vi "Lookup (Wfm Data Ref).vi"(8 "error in (no error)":errorcluster, 10 "Wfm Data Ref":T1, 11 "Reference Dictionary in":refnum<class "Reference Dictionary.lvclass">) -> (0 "error out":errorcluster, 1 "Index":i32, 2 "Found":bool, 3 "Reference Dictionary out":refnum<class "Reference Dictionary.lvclass">)   [LabVIEW 2015, in "Reference Dictionary.lvclass"]
uses:
  Reference Dictionary.lvclass
  <vilib>/NI Veristand/Custom Device API/Waveform Data Reference.ctl
  Reference Dictionary.lvclass/Reference Dictionary.ctl
  <vilib>/NI Veristand/Custom Device API/Custom Device API.lvlib
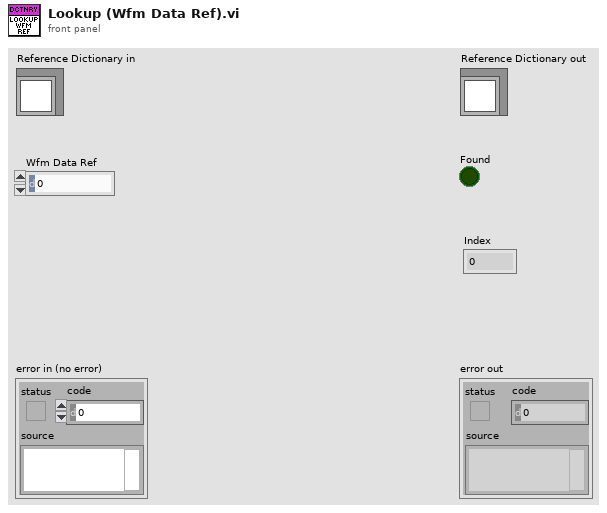
[diagram p1: front panel]
types:
  T1 = typedef "Custom Device API.lvlib/Waveform Data Reference.ctl" = i32
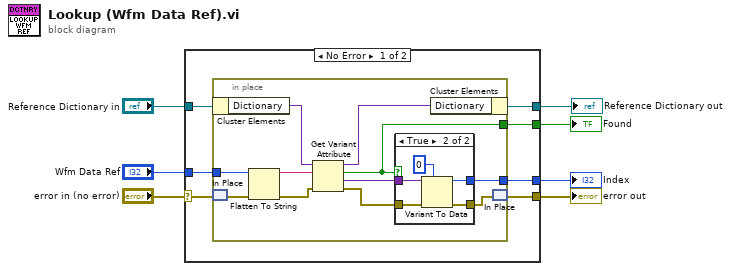
[diagram p0: block diagram]
diagram:
  n1 = case shown="No Error" "error in (no error)" {
    selector: "error in (no error)" -> [w14 w33]
    tunnel: [w13 w33] -> w6
    tunnel: [w9 w32] -> w4
    tunnel: "Reference Dictionary in" -> [w10 w32]
    tunnel: "Wfm Data Ref" -> [w12 _]
    tunnel: [w11 _] -> w2
    tunnel: [w8 _] -> w1
    frame No Error {
      n2 = in-place {
        in-place-border: w12 -> [w21]
        in-place-border: [w18] -> w11
        in-place-border: [w15] -> w8
        n3 = in-place-cluster #1(w10) -> ("Dictionary"=w22:variant)
        n4 = in-place-match #2(w14) -> (w23:errorcluster)
        n5 = Flatten To String(anything=w21, error in (no error)=w23) -> (data string=w25:string, error out=w20:errorcluster)  [unwired: 2 in, 1 out]
        n6 = Get Variant Attribute(Variant=w22, name=w25, error in=w20) -> (duplicate Variant=w16:variant, found=w15:bool, value=w24:variant, error out=w19:errorcluster)  [unwired: 1 in]
        n7 = case shown="True" w15 {
          tunnel: w24 -> [_ w31]
          tunnel: w19 -> [w26 w29]
          tunnel: [_ w28] -> w18
          tunnel: [w26 w27] -> w17
          frame False {
          }
          frame True {
            n8 = Variant To Data(error in=w29, type=0, Variant=w31) -> (data=w28:i32, error out=w27:errorcluster)
          }
        }
        n9 = in-place-cluster #1("Dictionary"=w16) -> (w9:refnum<class "Reference Dictionary.lvclass">)
        n10 = in-place-match #2(w17) -> (w13:errorcluster)
      }
    }
    frame Error {
    }
  }
  "error out" <- w6
  "Reference Dictionary out" <- w4
  "Index" <- w2
  "Found" <- w1
